vi "SCADA.vi"() -> ()   [LabVIEW 2024]
uses:
  <vilib>/Instr/_visa.llb/VISA Configure Serial Port (Instr).vi
  <vilib>/express/express arith-compare/Formula/XNode/ExpressFormulaBlockNode.xnode
panel:
  out "Erro Absoluto":dbl(graph)
  out "PWM":i32
  in  "Porta Serial":refnum<visa-resource-name>
  out "quente 2":bool
  out "Vento frio 2":bool
  out "Resistencia":bool
  out "Ventoinha":bool
  out "Temperatura ºC":dbl format="%.2f"
  out "Gráfico Temperatura e Set-Point":cluster{dbl, "Set-Point":dbl}(graph)
  in  "Set-Point":dbl
  out "Erros":errorcluster
  in  "STOP":bool
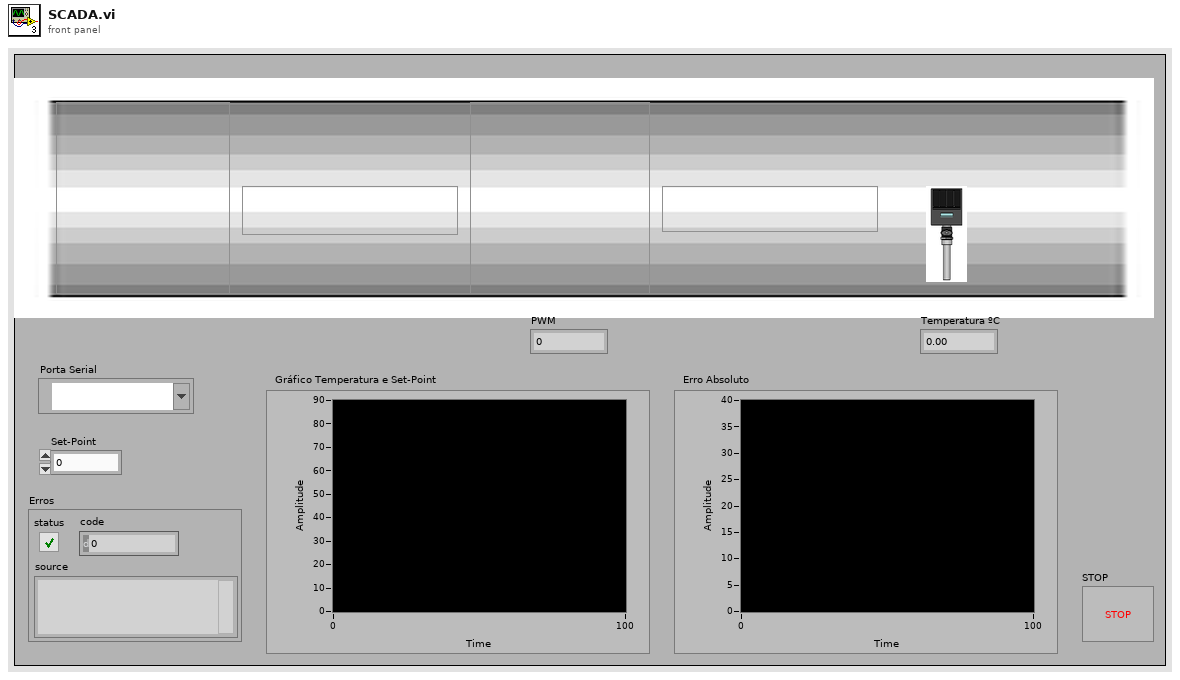
[diagram p1: front panel]
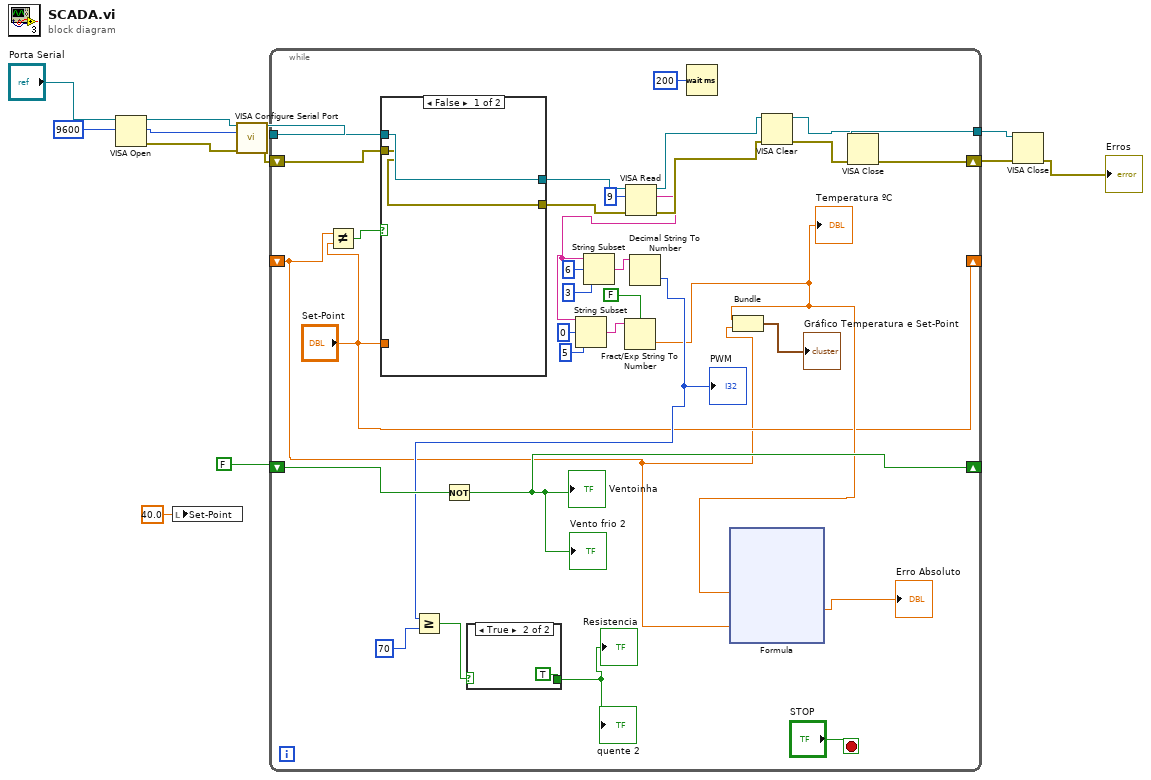
[diagram p0: block diagram]
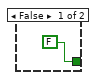
[diagram p2: hidden frame]
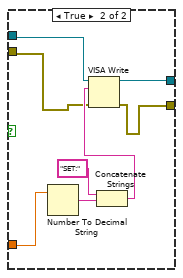
[diagram p3: hidden frame]
diagram:
  n1 = VISA Open(VISA resource name="Porta Serial") -> (VISA resource name=w7:refnum<visa-resource-name>, error out=w6:errorcluster)  [unwired: 4 in]
  n2 = local write "Set-Point"(40.0 ("Set-Point")) -> ()
  n3 = call-poly "VISA Configure Serial Port"("VISA resource name"=w7, "baud rate (9600)"=u32 9600, "error in (no error)"=w6) -> ("VISA resource name out"=w10:refnum<visa-resource-name>, "error out"=w9:errorcluster)  [unwired: 11 in]
  n4 = while {
    tunnel: w10 -> [w38]
    tunnel: [w33] -> w4
    shift-right: ["Set-Point"] -> _
    shift-left: _ -> [w12]
    shift-right: [w20] -> w3
    shift-left: w9 -> [w39]
    shift-right: [w30] -> _
    shift-left: FALSE -> [w31]
    stop <- "STOP" stop-if-true
    n5 = Not Equal?(x=w12, y="Set-Point") -> (x != y?=w35:bool)
    n6 = case shown="False" w35 {
      tunnel: "Set-Point" -> [_ w61]
      tunnel: [w55 w60] -> w41
      tunnel: [w56 w59] -> w40
      tunnel: w39 -> [w55 w58]
      tunnel: w38 -> [w56 w57]
      frame False {
      }
      frame True {
        n7 = Number To Decimal String(number=w61) -> (decimal integer string=w64:string)  [unwired: 1 in]
        n8 = Concatenate Strings("SET:" ("string"), w64) -> (w62:string)
        n9 = VISA Write(VISA resource name=w57, write buffer=w62, error in (no error)=w58) -> (VISA resource name out=w59:refnum<visa-resource-name>, error out=w60:errorcluster)  [unwired: 1 out]
      }
    }
    n10 = Not(x=w31) -> (.not. x?=w30:bool)
    "Ventoinha" <- w30
    "Vento frio 2" <- w30
    n11 = VISA Read(VISA resource name=w40, byte count=u32 9, error in (no error)=w41) -> (VISA resource name out=w34:refnum<visa-resource-name>, read buffer=w14:string, error out=w32:errorcluster)  [unwired: 1 out]
    n12 = String Subset(string=w14, offset (0)=0, length (rest)=5 ("length (rest)")) -> (substring=w16:string)
    n13 = String Subset(string=w14, offset (0)=6, length (rest)=3 ("length (rest)")) -> (substring=w15:string)
    n14 = Fract/Exp String To Number(use system decimal point (T)=FALSE, string=w16) -> (number=w17:dbl)  [unwired: 2 in, 1 out]
    "Temperatura ºC" <- w17
    n15 = Decimal String To Number(string=w15) -> (number=w19:i32)  [unwired: 2 in, 1 out]
    "PWM" <- w19
    n16 = Greater Or Equal?(x=w19, y=70) -> (x >= y?=w28:bool)
    n17 = case shown="True" w28 {
      tunnel: [FALSE TRUE] -> w27
      frame False {
      }
      frame True {
      }
    }
    "quente 2" <- w27
    "Resistencia" <- w27
    n18 = Wait (ms)(milliseconds to wait=u32 200) -> ()  [unwired: 1 out]
    n19 = xnode "Formula"("X1"=w17, "X2"=w12) -> ("Result"=→"Erro Absoluto":dbl)  [unwired: 1 in, 1 out]
    n20 = Bundle(w17, "Set-Point"=w12) -> (→"Gráfico Temperatura e Set-Point":cluster{dbl, "Set-Point":dbl})  [unwired: 1 in]
    n21 = VISA Clear(VISA resource name=w34, error in (no error)=w32) -> (VISA resource name out=w33:refnum<visa-resource-name>, error out=w20:errorcluster)
  }
  n22 = VISA Close(VISA resource name=w4, error in (no error)=w3) -> ()  [unwired: 1 out]
  n23 = VISA Close(VISA resource name=w4, error in (no error)=w3) -> (error out=→"Erros":errorcluster)
